vi "K6514_ReadCharge.vi"(0 "VISA resource name":refnum<visa-resource-name>, 5 "position":string, 7 "Number of Pulses":i32, 9 "Laser Energy (uJ)":dbl, 11 "error in (no error)":errorcluster, 12 "file refnum":refnum<file>) -> (4 "VISA resource name out":refnum<visa-resource-name>, 6 "charge(C)":dbl, 10 "Response":string, 14 "file refnum out":refnum<file>, 15 "error out":errorcluster)   [LabVIEW 2024]
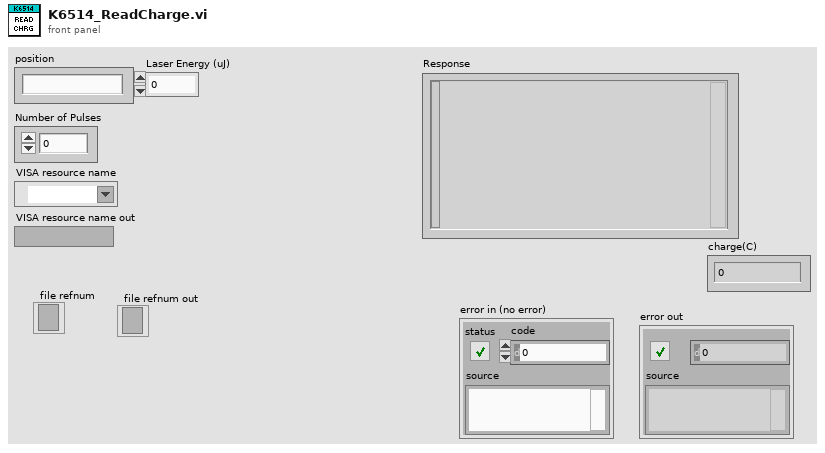
[diagram p1: front panel]
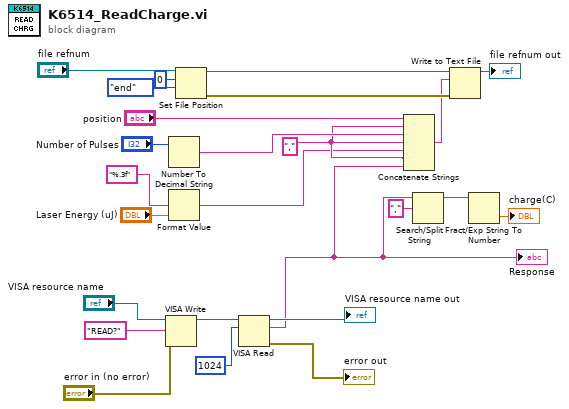
[diagram p0: block diagram]
diagram:
  w4 = "," ("string")
  n1 = VISA Write(VISA resource name="VISA resource name", write buffer="READ?" ("String"), error in (no error)="error in (no error)") -> (VISA resource name out=w22:refnum<visa-resource-name>)  [unwired: 2 out]
  n2 = Number To Decimal String(number="Number of Pulses") -> (decimal integer string=w13:string)  [unwired: 1 in]
  n3 = Format Value(format string="%.3f", value (0)="Laser Energy (uJ)") -> (output string=w1:string)  [unwired: 1 in]
  n4 = Set File Position(offset (in bytes) (0)=i64 0, refnum="file refnum", from (0:start)=enum16{"start", "end", "current"}."end") -> (refnum out=w18:refnum<file>, error out=w21:errorcluster)  [unwired: 1 in]
  n5 = VISA Read(VISA resource name=w22, byte count=u32 1024 ("Read Count")) -> (VISA resource name out=→"VISA resource name out":refnum<visa-resource-name>, read buffer=w5:string, error out=→"error out":errorcluster)  [unwired: 1 in, 1 out]
  "Response" <- w5
  n6 = Concatenate Strings("position", w4, w13, w4, w1, w4, w5) -> (w15:string)
  n7 = Search/Split String(string=w5, search string/char (-)=",") -> (substring before match=w10:string)  [unwired: 1 in, 2 out]
  n8 = Write to Text File(file (use dialog)=w18, text=w15, error in=w21) -> (refnum out=→"file refnum out":refnum<file>)  [unwired: 1 in, 2 out]
  n9 = Fract/Exp String To Number(string=w10) -> (number=→"charge(C)":dbl)  [unwired: 3 in, 1 out]
